vi "EncodeSignedHundredths.vi"(1 "Data In":dbl[](array[numeric])) -> (0 "Data Out":u8[](array[numeric]))   [LabVIEW 2015, in "navX Library v1 (deprecated).lvlib"]
uses:
  navX Library v1 (deprecated).lvlib
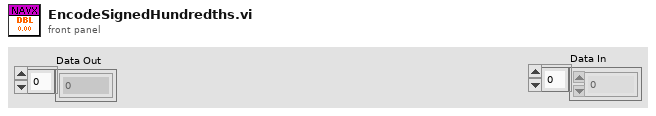
[diagram p1: front panel]
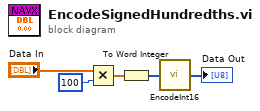
[diagram p0: block diagram]
diagram:
  n1 = Multiply(x="Data In", y=100) -> (x*y=w3:dbl[])
  n2 = To Word Integer(number=w3) -> (16bit integer=w1:i16[])
  n3 = call "EncodeInt16.vi"("Data In"=w1) -> ("Data Out"=→"Data Out":u8[])
